vi "ICM Locate Analog Phys Channels.vi"(0 "Channel Type":enum16{"AD SE", "AD Diff", "DA"}(ring), 11 "error in (no error)":errorcluster) -> (4 "Table":string[][](table), 15 "error out":errorcluster)   [LabVIEW 2024]
doc: "MICAS Locate Analog Phys Channels.vi\n\nThis VI scans connected NI DAQ devices for the type of analog channel specified by Channel Type. It returns a table indicating the number of channels of the specified type for each connected device."
uses:
  C:/Program Files/NI/LVAddons/nidaqmx/1/resource/objmgr/daqmx.rc
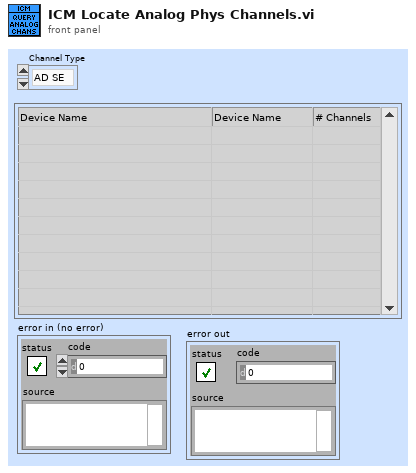
[diagram p1: front panel]
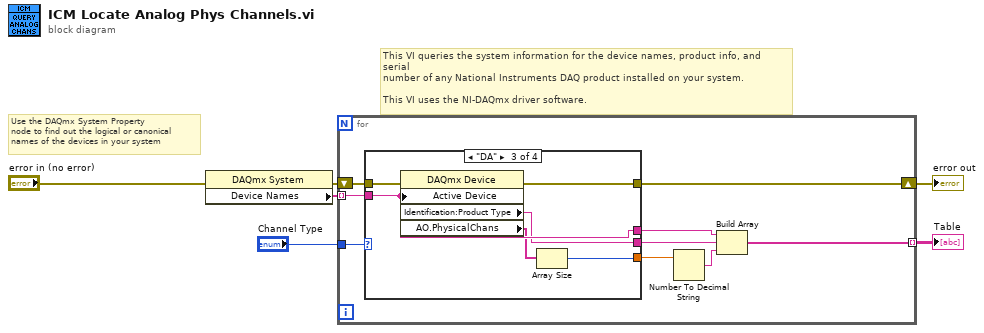
[diagram p0: block diagram]
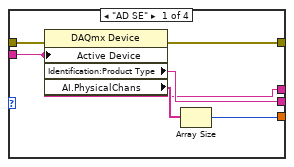
[diagram p2: hidden frame]
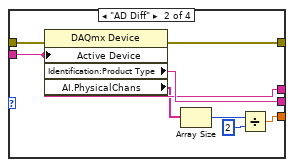
[diagram p3: hidden frame]
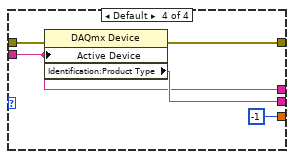
[diagram p4: hidden frame]
diagram:
  # "This VI queries the system information for the device names, product info, and serial \nnumber of any National Instruments DAQ product installed on your system.\n\nThis VI uses the NI-DAQmx driver software."
  # "Use the DAQmx System Property\nnode to find out the logical or canonical\nnames of the devices in your system"
  n1 = property class="DAQmx System"(error in="error in (no error)") -> (error out=w6:errorcluster, "Device Names"=w5:tag[])  [unwired: 1 in, 1 out]
  n2 = for {
    tunnel: w5 -> [w14] mode=indexing
    shift-right: [w9] -> w3
    shift-left: w6 -> [w10]
    tunnel: "Channel Type" -> [w15]
    tunnel: [w8] -> w1 mode=indexing
    n3 = case shown="\"DA\"" w15 {
      tunnel: w14 -> [w17 w28 w35 w39]
      tunnel: [w18 w22 w30 -1] -> w7
      tunnel: [w19 w29 w34 w40] -> w13
      tunnel: [w17 w28 w35 w39] -> w11
      tunnel: w10 -> [w16 w27 w33 w38]
      tunnel: [w20 w26 w32 w37] -> w9
      frame "AD SE" {
        n4 = property class="DAQmx Device"(error in=w16, "Active Device"=w17) -> (error out=w20:errorcluster, "Identification:Product Type"=w19:string, "AI.PhysicalChans"=w21:tag[])  [unwired: 1 in, 1 out]
        n5 = Array Size(array=w21) -> (size(s)=w18:i32)
      }
      frame "AD Diff" {
        n6 = property class="DAQmx Device"(error in=w27, "Active Device"=w28) -> (error out=w26:errorcluster, "Identification:Product Type"=w29:string, "AI.PhysicalChans"=w25:tag[])  [unwired: 1 in, 1 out]
        n7 = Array Size(array=w25) -> (size(s)=w24:i32)
        n8 = Divide(x=w24, y=2) -> (x/y=w22:dbl)
      }
      frame "DA" {
        n9 = property class="DAQmx Device"(error in=w33, "Active Device"=w35) -> (error out=w32:errorcluster, "Identification:Product Type"=w34:string, "AO.PhysicalChans"=w31:tag[])  [unwired: 1 in, 1 out]
        n10 = Array Size(array=w31) -> (size(s)=w30:i32)
      }
      frame Default {
        n11 = property class="DAQmx Device"(error in=w38, "Active Device"=w39) -> (error out=w37:errorcluster, "Identification:Product Type"=w40:string)  [unwired: 1 in, 1 out]
      }
    }
    n12 = Number To Decimal String(number=w7) -> (decimal integer string=w12:string)  [unwired: 1 in]
    n13 = Build Array(w11, w13, w12) -> (w8:string[])
  }
  "Table" <- w1
  "error out" <- w3
